vi "Initialize.vi"(8 "error in (no error)":errorcluster, 11 "VISA resource name":refnum<visa-resource-name>) -> (0 "error out":errorcluster, 3 "VISA resource name out":refnum<visa-resource-name>, 4 "Device Errors":cluster{"code":i32, "Text":string}[](array[cluster]))   [LabVIEW 2014, in "Stanford Research DG645 - Driver.lvlib"]
doc: "Establishes communication with the instrument. Therefore, call this VI before calling other instrument driver VIs for this instrument. Generally, you need to call the Initialize VI only once at the beginning of an application."
uses:
  Stanford Research DG645 - Driver.lvlib
panel:
  # "(c) 2012 GSI Helmholtzzentrum für Schwerionenforschung GmbH.  ALL RIGHTS RESERVED."
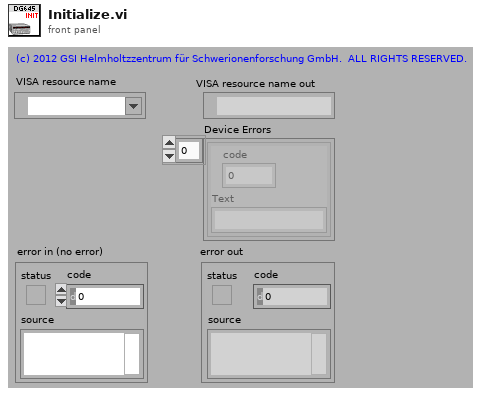
[diagram p1: front panel]
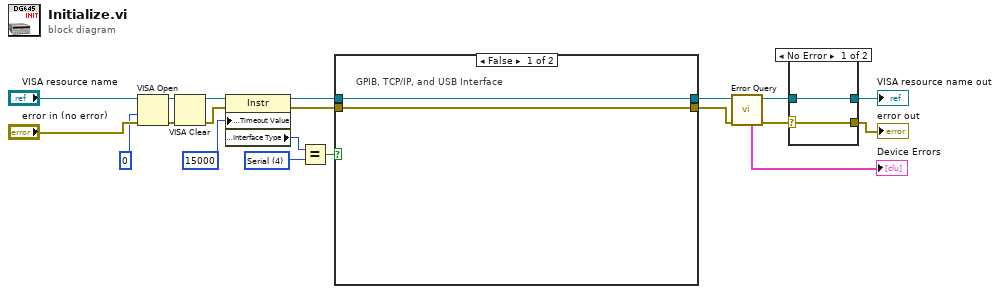
[diagram p0: block diagram]
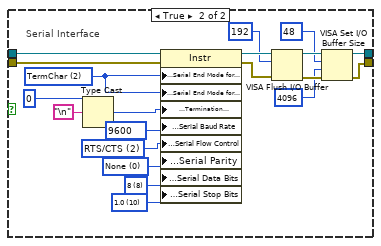
[diagram p2: hidden frame]
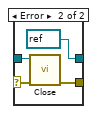
[diagram p3: hidden frame]
diagram:
  w13 = u16 4 items=["GPIB"=1, "VXI"=2, "GPIB-VXI"=3, "Serial"=4, "PXI"=5, "TCPIP"=6, "USB"=7] ("Interface Information:Interface Type")
  n1 = VISA Open(access mode=u32 0, error in (no error)="error in (no error)", VISA resource name="VISA resource name") -> (VISA resource name=w11:refnum<visa-resource-name>, error out=w10:errorcluster)  [unwired: 2 in]
  n2 = VISA Clear(VISA resource name=w11, error in (no error)=w10) -> (VISA resource name out=w9:refnum<visa-resource-name>, error out=w8:errorcluster)
  n3 = property class="Instr"(reference=w9, error in=w8, "General Settings:Timeout Value"=u32 15000) -> (reference out=w16:refnum<visa-resource-name>, error out=w15:errorcluster, "Interface Information:Interface Type"=w18:u16)
  n4 = Equal?(x=w18, y=w13) -> (x = y?=w14:bool)
  n5 = case shown="False" w14 {
    tunnel: [w21 w39] -> w3
    tunnel: [w22 w36] -> w2
    tunnel: w16 -> [w21 w41]
    tunnel: w15 -> [w22 w42]
    frame False {
      # "GPIB, TCP/IP, and USB Interface"
    }
    frame True {
      w23 = u16 10 items=["1.0"=10, "1.5"=15, "2.0"=20] ("Stop Bits")
      w24 = u16 8 items=["7"=7, "8"=8] ("Data Bits")
      w25 = u16 0 items=["None", "Odd", "Even", "Mark", "Space"] ("Serial Settings:Parity")
      w26 = u16 2 items=["None", "XON/XOFF", "RTS/CTS", "XON/XOFF & RTS/CTS", "DTR/DSR", "XON/XOFF & DTR/DSR"] ("Serial Settings:Flow Control")
      w27 = u32 9600 items=["300"=300, "600"=600, "1200"=1200, "2400"=2400, "4800"=4800, "9600"=9600, "19200"=19200] ("Baud Rate")
      w29 = u16 2 items=["None", "LastBit", "TermChar"] ("Serial Settings:Serial End Mode for Reads")
      # "Serial Interface"
      n6 = Type Cast(type=u8 0, x="\n" ("Line Feed Constant")) -> (*(type *) &x=w28:u8)
      n7 = property class="Instr"(reference=w41, error in=w42, "Serial Settings:Serial End Mode for Reads"=w29, "Serial Settings:Serial End Mode for Writes"=w29, "Message Based Settings:Termination Character"=w28, "Serial Settings:Serial Baud Rate"=w27, "Serial Settings:Serial Flow Control"=w26, "Serial Settings:Serial Parity"=w25, "Serial Settings:Serial Data Bits"=w24, "Serial Settings:Serial Stop Bits"=w23) -> (reference out=w35:refnum<visa-resource-name>, error out=w38:errorcluster)
      n8 = VISA Flush I/O Buffer(VISA resource name=w35, mask (16)=u16 192, error in (no error)=w38) -> (VISA resource name out=w40:refnum<visa-resource-name>, error out=w37:errorcluster)
      n9 = VISA Set I/O Buffer Size(VISA resource name=w40, mask (16)=u16 48, size (4096)=u32 4096 ("size (0)"), error in (no error)=w37) -> (VISA resource name out=w39:refnum<visa-resource-name>, error out=w36:errorcluster)
    }
  }
  n10 = call "Error Query.vi"("error in (no error)"=w2, "VISA resource name"=w3) -> ("error out"=w1:errorcluster, "VISA resource name out"=w5:refnum<visa-resource-name>, "Device Errors"=→"Device Errors":cluster{"code":i32, "Text":string}[])  [unwired: 7 in]
  n11 = case shown="No Error" w1 {
    selector: w1 -> [w43 w46]
    tunnel: w5 -> [w44 w47]
    tunnel: [w44 refnum<visa-resource-name> refnum ("VISA resource name out")] -> w7
    tunnel: [w43 w48] -> w6
    frame No Error {
    }
    frame Error {
      n12 = call "Close.vi"("error in (no error)"=w46, "VISA resource name"=w47) -> ("error out"=w48:errorcluster)  [unwired: 8 in, 1 out]
    }
  }
  "VISA resource name out" <- w7
  "error out" <- w6
